vi "Wojtek control.vi"(9 "Desired Angle":dbl format="%#_13g", 10 "Gyro Angle":dbl format="%#_13g", 11 "Speed":dbl format="%#_13g") -> (2 "right axis value":dbl=-0.4793390142671308, 3 "left axis value":dbl=-0.5206609857328692)   [LabVIEW 2015]
panel:
  in  "kp":dbl=0.02
  in  "kd":dbl=0.0015
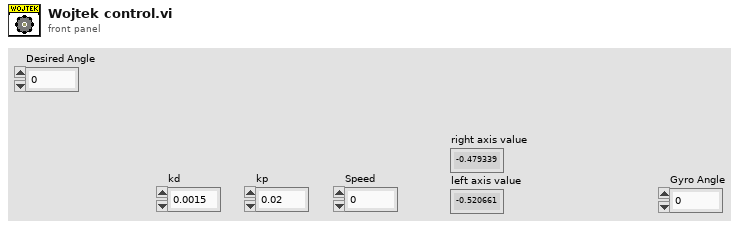
[diagram p1: front panel]
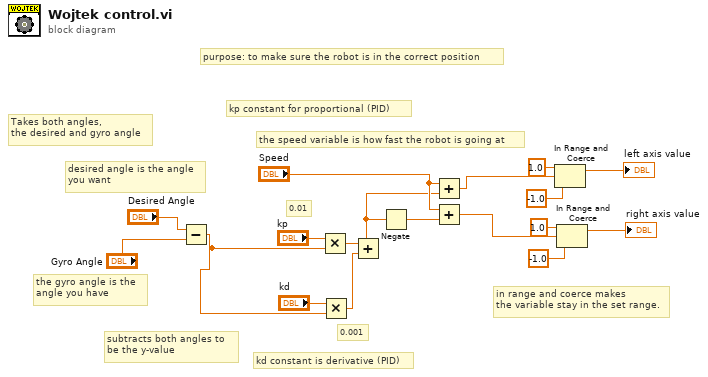
[diagram p0: block diagram]
diagram:
  # "purpose: to make sure the robot is in the correct position"
  # "the speed variable is how fast the robot is going at"
  # "kd constant is derivative (PID)"
  # "in range and coerce makes\nthe variable stay in the set range."
  # "kp constant for proportional (PID)"
  # "subtracts both angles to \nbe the y-value"
  # "the gyro angle is the \nangle you have"
  # "desired angle is the angle \nyou want"
  # "Takes both angles, \nthe desired and gyro angle"
  # "0.01"
  # "0.001"
  n1 = Subtract(x="Desired Angle", y="Gyro Angle") -> (x-y=w1:dbl)
  n2 = Multiply(x="kp", y=w1) -> (x*y=w18:dbl)
  n3 = Multiply(x="kd", y=w1) -> (x*y=w17:dbl)
  n4 = Add(x=w18, y=w17) -> (x+y=w5:dbl)
  n5 = Negate(x=w5) -> (-x=w4:dbl)
  n6 = Add(x="Speed", y=w5) -> (x+y=w10:dbl)
  n7 = Add(x="Speed", y=w4) -> (x+y=w14:dbl)
  n8 = In Range and Coerce(upper limit=1.0, x=w10, lower limit=-1.0) -> (coerced(x)=→"left axis value":dbl)  [unwired: 1 out]
  n9 = In Range and Coerce(upper limit=1.0, x=w14, lower limit=-1.0) -> (coerced(x)=→"right axis value":dbl)  [unwired: 1 out]
